vi "ACTUATOR ENC.vi"() -> (1 "RIGHT ACT POS":fxp<+,51,11>, 2 "LEFT ACT POS":fxp<+,51,11>)   [LabVIEW 2019]
uses:
  <vilib>/Platform/TimedLoop/XDataNode/timing_clust.ctl
  <vilib>/Platform/TimedLoop/XDataNode/nitl_modes.ctl
  <vilib>/Platform/TimedLoop/XDataNode/wakeup.ctl
  <vilib>/rvi/Emulation/niFpgaSctlEmulationGetInTimedLoop.vi
  <vilib>/rvi/Emulation/niFpgaEmulationReportErrorSimple.vi
  <vilib>/rvi/Emulation/niFpgaGetClockAttributes.vi
  <vilib>/rvi/Emulation/niFpgaCriticalErrorInLSC.vi
  <vilib>/rvi/eio/common/nirviEmuTemplateMethod_errors.vi
  <vilib>/platform/TimedLoop/XDataNode/XDataNode.xnode
  <vilib>/eio/EIONode/EIONode.xnode
  <vilib>/Platform/TimedLoop/XDataNode/XDNodeRunTimeDep.lvlib
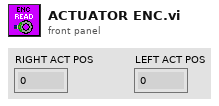
[diagram p1: front panel]
types:
  T1 = typedef "XDNodeRunTimeDep.lvlib/timing_clust.ctl" = cluster{"Expected End [f-1]":u64, "Actual End [f-1]":u64, "Finished Late? [f-1]":bool, "Expected End [i-1]":u64, "Actual End [i-1]":u64, "Finished Late? [i-1]":bool, "Expected Start [i]":u64, "Actual Start [i]":u64, "Expected Start [f]":u64, "Actual Start [f]":u64, "Source Name":string, "Structure Name":string, "Period":i64, "Deadline":i64, "Offset":i64, "Start":i64, "Priority":i32, "Timeout":i32, "Mode":T2, "Wakeup Reason":T3, "Error":errorcluster, "Source Type":string, "Secondary Source Type":string, "Global End Time":u64, "Global Start Time":u64, "Frame Duration":u64, "Iteration Duration":u64, "Assigned CPU":i32, "I/O Scan Engine Mode":u32}
  T2 = typedef "XDNodeRunTimeDep.lvlib/nitl_modes.ctl" = enum32{"No Change", "Process missed periods, maintain original phase", "Discard missed periods, maintain original phase", "Process missed periods, ignore original phase", "Discard missed periods, ignore original phase"}
  T3 = typedef "XDNodeRunTimeDep.lvlib/wakeup.ctl" = enum32{"Normal", "Aborted", "Asynchronous wakeup", "Timing source error", "Timed loop error", "Timeout"}
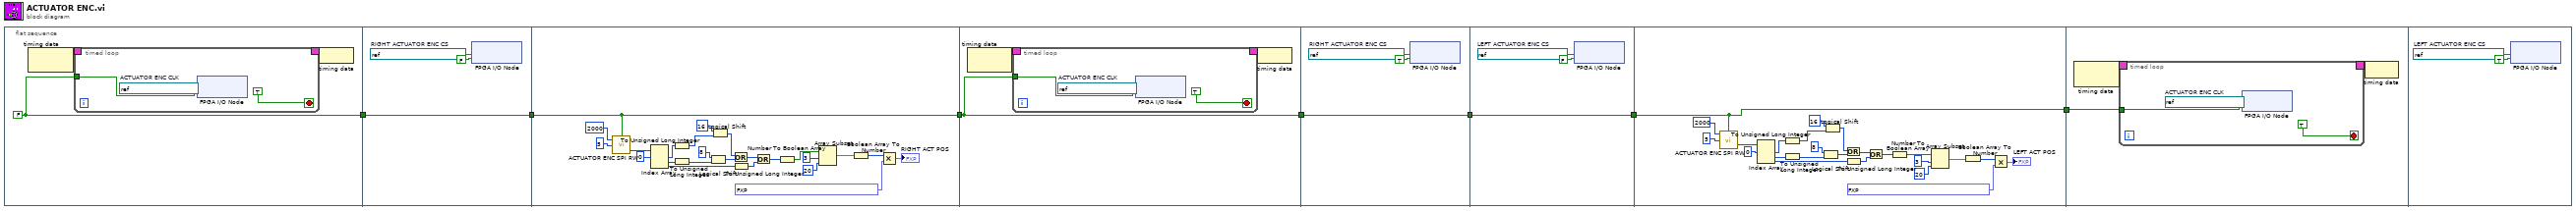
[diagram p0: block diagram]
diagram:
  n1 = flat-sequence {
    tunnel: [w8] -> w7
    tunnel: [w20] -> w6
    tunnel: w7 -> [w20]
    tunnel: w6 -> [w44]
    tunnel: [w44] -> w5
    tunnel: w5 -> [w45]
    tunnel: [w45] -> w4
    tunnel: w4 -> [w55]
    tunnel: [w55] -> w3
    tunnel: w3 -> [w58]
    tunnel: [w58] -> w2
    tunnel: w2 -> [w61]
    tunnel: [w61] -> w1
    tunnel: w1 -> [w85]
    frame #0 {
      w8 = FALSE ("CPOL")
      n2 = node-c288() -> (w10:T1)  [unwired: 1 in]
      n3 = timed-loop {
        timing: w10 -> [_]
        timing-out: [_] -> w9
        tunnel: w8 -> [w12]
        stop <- TRUE stop-if-true
        w11 = refnum<k21> "ACTUATOR ENC CLK"  # ACTUATOR ENC CLK
        n4 = xnode "FPGA I/O Node"("I/O Item"=w12, "FPGA I/O In"=w11) -> ()  [unwired: 1 out]
      }
      n5 = node-c288(w9) -> ()
    }
    frame #1 {
      w19 = refnum<k21> "RIGHT ACTUATOR ENC CS"  # RIGHT ACTUATOR ENC CS
      n6 = xnode "FPGA I/O Node"("I/O Item"=FALSE ("Value"), "FPGA I/O In"=w19) -> ()  [unwired: 1 out]
    }
    frame #2 {
      n7 = call "ACTUATOR ENC SPI RW.vi"("CPOL"=w44, "Frames to Write"=u8 5, "SPI Frequency (KHz)"=u16 2000 ("Frequency (kHz)")) -> ("Data Read"=w22:u8[])  [unwired: 1 in, 1 out]
      n8 = Index Array(array=w22, index #1=0 ("index")) -> (element #1=w29:u8, element #2=w36:u8, element #3=w37:u8)  [unwired: 2 in]
      n9 = To Unsigned Long Integer(number=w29) -> (unsigned 32bit integer=w30:u32)
      n10 = To Unsigned Long Integer(number=w36) -> (unsigned 32bit integer=w31:u32)
      n11 = Logical Shift(y=i16 8, x=w31) -> (x << y=w33:u32)
      n12 = Logical Shift(y=i16 16, x=w30) -> (x << y=w32:u32)
      n13 = Or(x=w32, y=w33) -> (x .or. y?=w34:u32)
      n14 = To Unsigned Long Integer(number=w37) -> (unsigned 32bit integer=w35:u32)
      n15 = Or(x=w34, y=w35) -> (x .or. y?=w42:u32)
      n16 = Number To Boolean Array(number=w42) -> (Boolean array=w38:bool[])
      n17 = Array Subset(array=w38, index=3, length=20) -> (w39:bool[])
      n18 = Boolean Array To Number(Boolean array=w39) -> (number=w40:u32)
      n19 = Multiply(x=w40, y=fxp<+,28,-11> 0.00034332307950535323) -> (x*y=→"RIGHT ACT POS":fxp<+,60,21>)
    }
    frame #3 {
      n20 = node-c288() -> (w47:T1)  [unwired: 1 in]
      n21 = timed-loop {
        timing: w47 -> [_]
        timing-out: [_] -> w46
        tunnel: w45 -> [w49]
        stop <- TRUE stop-if-true
        w48 = refnum<k21> "ACTUATOR ENC CLK"  # ACTUATOR ENC CLK
        n22 = xnode "FPGA I/O Node"("I/O Item"=w49, "FPGA I/O In"=w48) -> ()  [unwired: 1 out]
      }
      n23 = node-c288(w46) -> ()
    }
    frame #4 {
      w57 = refnum<k21> "RIGHT ACTUATOR ENC CS"  # RIGHT ACTUATOR ENC CS
      n24 = xnode "FPGA I/O Node"("I/O Item"=TRUE ("Value"), "FPGA I/O In"=w57) -> ()  [unwired: 1 out]
    }
    frame #5 {
      w60 = refnum<k21> "LEFT ACTUATOR ENC CS"  # LEFT ACTUATOR ENC CS
      n25 = xnode "FPGA I/O Node"("I/O Item"=FALSE ("Value"), "FPGA I/O In"=w60) -> ()  [unwired: 1 out]
    }
    frame #6 {
      n26 = call "ACTUATOR ENC SPI RW.vi"("CPOL"=w61, "Frames to Write"=u8 5, "SPI Frequency (KHz)"=u16 2000 ("Frequency (kHz)")) -> ("Data Read"=w63:u8[])  [unwired: 1 in, 1 out]
      n27 = Index Array(array=w63, index #1=0 ("index")) -> (element #1=w70:u8, element #2=w77:u8, element #3=w78:u8)  [unwired: 2 in]
      n28 = To Unsigned Long Integer(number=w70) -> (unsigned 32bit integer=w71:u32)
      n29 = To Unsigned Long Integer(number=w77) -> (unsigned 32bit integer=w72:u32)
      n30 = Logical Shift(y=i16 8, x=w72) -> (x << y=w74:u32)
      n31 = Logical Shift(y=i16 16, x=w71) -> (x << y=w73:u32)
      n32 = Or(x=w73, y=w74) -> (x .or. y?=w75:u32)
      n33 = To Unsigned Long Integer(number=w78) -> (unsigned 32bit integer=w76:u32)
      n34 = Or(x=w75, y=w76) -> (x .or. y?=w83:u32)
      n35 = Number To Boolean Array(number=w83) -> (Boolean array=w79:bool[])
      n36 = Array Subset(array=w79, index=3, length=20) -> (w80:bool[])
      n37 = Boolean Array To Number(Boolean array=w80) -> (number=w81:u32)
      n38 = Multiply(x=w81, y=fxp<+,28,-11> 0.00034332307950535323) -> (x*y=→"LEFT ACT POS":fxp<+,60,21>)
    }
    frame #7 {
      n39 = node-c288() -> (w87:T1)  [unwired: 1 in]
      n40 = timed-loop {
        timing: w87 -> [_]
        timing-out: [_] -> w86
        tunnel: w85 -> [w89]
        stop <- TRUE stop-if-true
        w88 = refnum<k21> "ACTUATOR ENC CLK"  # ACTUATOR ENC CLK
        n41 = xnode "FPGA I/O Node"("I/O Item"=w89, "FPGA I/O In"=w88) -> ()  [unwired: 1 out]
      }
      n42 = node-c288(w86) -> ()
    }
    frame #8 {
      w96 = refnum<k21> "LEFT ACTUATOR ENC CS"  # LEFT ACTUATOR ENC CS
      n43 = xnode "FPGA I/O Node"("I/O Item"=TRUE ("Value"), "FPGA I/O In"=w96) -> ()  [unwired: 1 out]
    }
  }
